vi "co-pilot teleop recieve.vi"(9 "MechanismMetrics in":T1, 10 "empty?":bool, 11 "Co-Pilot Data in":T4) -> (2 "MechanismMetrics out":T1)   [LabVIEW 2014]
uses:
  Lifter Hights.vi
  Lifter States.ctl
  MechanismMetrics.ctl
  Co-Pilot_game_control.ctl
  Auto Lifter States.ctl
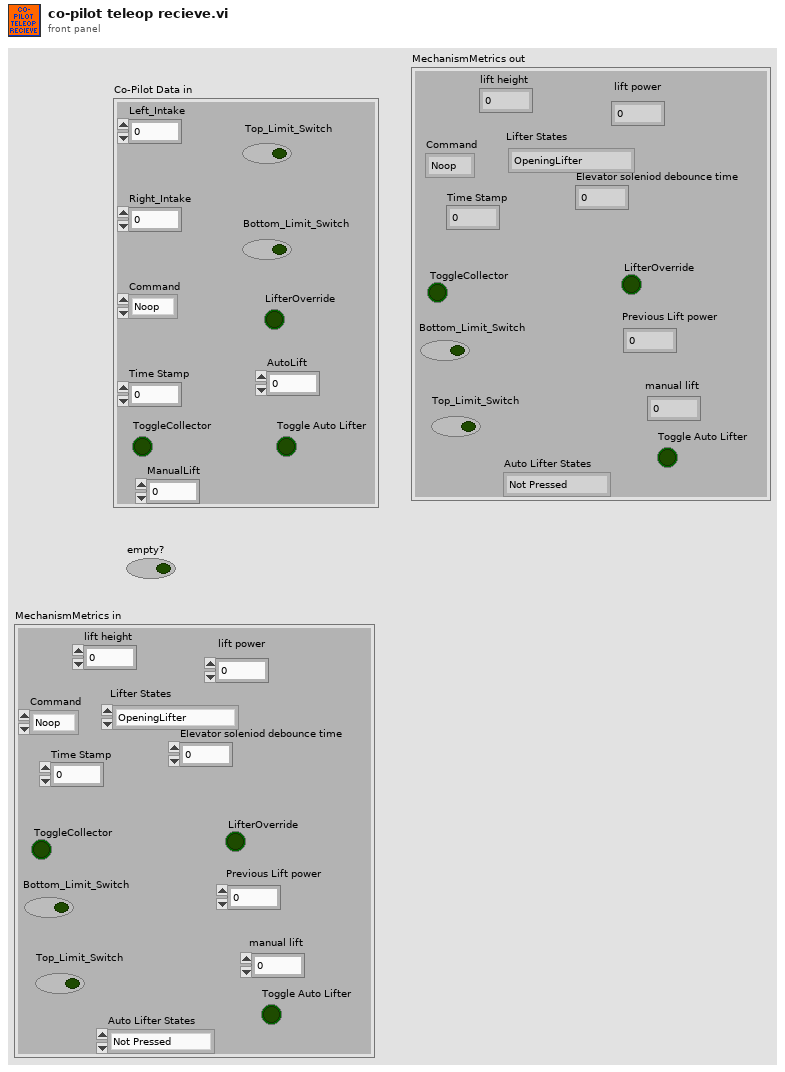
[diagram p1: front panel]
types:
  T1 = typedef "MechanismMetrics.ctl" = cluster{"lift height":dbl, "Command":enum16{"Noop", "Flagged"}, "Time Stamp":u32, "ToggleCollector":bool, "Bottom_Limit_Switch ":bool, "Top_Limit_Switch":bool, "lift power":dbl, "Elevator soleniod debounce time   ":dbl, "LifterOverride":bool, "Previous Lift power":dbl, "manual lift":dbl, "Lifter States":T2, "Auto Lifter States":T3, "Toggle Auto Lifter":bool}
  T2 = typedef "Lifter States.ctl" = enum16{"OpeningLifter", "LifterOpen", "ClosingLifter", "LifterClosed"}
  T3 = typedef "Auto Lifter States.ctl" = enum16{"Not Pressed", "Press Detected", "To Setpoint 1", "To Setpoint 2", "Open Lifter", "Close", "To Setpoint 3"}
  T4 = typedef "Co-Pilot_game_control.ctl" = cluster{"Left_Intake":dbl, "Right_Intake":dbl, "Time Stamp":u32, "Command":enum16{"Noop", "Flagged"}, "ToggleCollector":bool, "ManualLift":dbl, "Top_Limit_Switch":bool, "Bottom_Limit_Switch ":bool, "LifterOverride":bool, "AutoLift":i32, "Toggle Auto Lifter":bool}
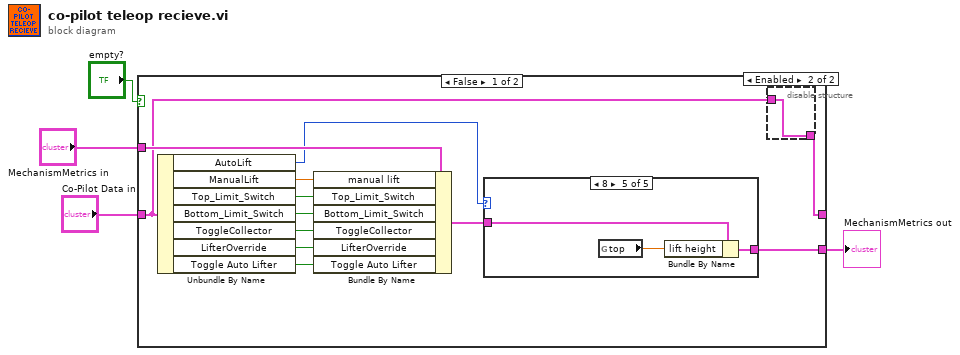
[diagram p0: block diagram]
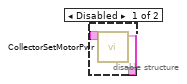
[diagram p2: hidden frame]
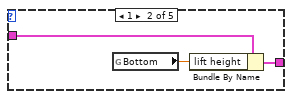
[diagram p4: hidden frame]
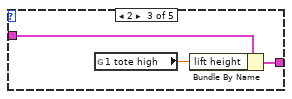
[diagram p5: hidden frame]
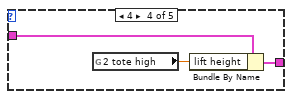
[diagram p6: hidden frame]
diagram:
  n1 = case shown="False" "empty?" {
    tunnel: "Co-Pilot Data in" -> [w14 w34]
    tunnel: [w16 w34] -> _
    tunnel: "MechanismMetrics in" -> [w15 w33]
    tunnel: [w9 w33] -> w1
    frame False {
      n2 = Unbundle By Name(w14) -> ("AutoLift"=w7:i32, "ManualLift"=w6:dbl, "Top_Limit_Switch"=w13:bool, "Bottom_Limit_Switch"=w12:bool, "ToggleCollector"=w11:bool, "LifterOverride"=w8:bool, "Toggle Auto Lifter"=w5:bool)
      n3 = Bundle By Name(cluster=w15, "manual lift"=w6, "Top_Limit_Switch"=w13, "Bottom_Limit_Switch"=w12, "ToggleCollector"=w11, "LifterOverride"=w8, "Toggle Auto Lifter"=w5) -> (w10:T1)
      n4 = case shown="8" w7 {
        tunnel: [w20 w23 w26 w29 w32] -> w9
        tunnel: w10 -> [w20 w21 w24 w27 w30]
        frame 0, Default {
        }
        frame 1 {
          n5 = global read "Lifter Hights.vi" "Bottom"() -> (w22:dbl)
          n6 = Bundle By Name(cluster=w21, "lift height"=w22) -> (w23:T1)
        }
        frame 2 {
          n7 = global read "Lifter Hights.vi" "1 tote high"() -> (w25:dbl)
          n8 = Bundle By Name(cluster=w24, "lift height"=w25) -> (w26:T1)
        }
        frame 4 {
          n9 = global read "Lifter Hights.vi" "2 tote high"() -> (w28:dbl)
          n10 = Bundle By Name(cluster=w27, "lift height"=w28) -> (w29:T1)
        }
        frame 8 {
          n11 = global read "Lifter Hights.vi" "top"() -> (w31:dbl)
          n12 = Bundle By Name(cluster=w30, "lift height"=w31) -> (w32:T1)
        }
      }
      n13 = disable-structure shown="Enabled" {
        disable-tunnel: [w18 w19] -> w16
        disable-tunnel: w14 -> [w17 w19]
        frame Disabled {
          n14 = call "CollectorSetMotorPwr.vi"("Co-Pilot Data in"=w17) -> ("Co-Pilot Data out"=w18:T4)  [unwired: 10 in]
        }
        frame Enabled {
        }
      }
    }
    frame True {
    }
  }
  "MechanismMetrics out" <- w1
